vi "Apply Surface.vi"(5 "x":i32, 7 "y":i32, 8 "error in":errorcluster, 10 "Destination Pointer":u32, 11 "Source Pointer":u32) -> (0 "error out":errorcluster)   [LabVIEW 2015]
uses:
  Controls/Rectangle.ctl
  LibSDL2.lvlib
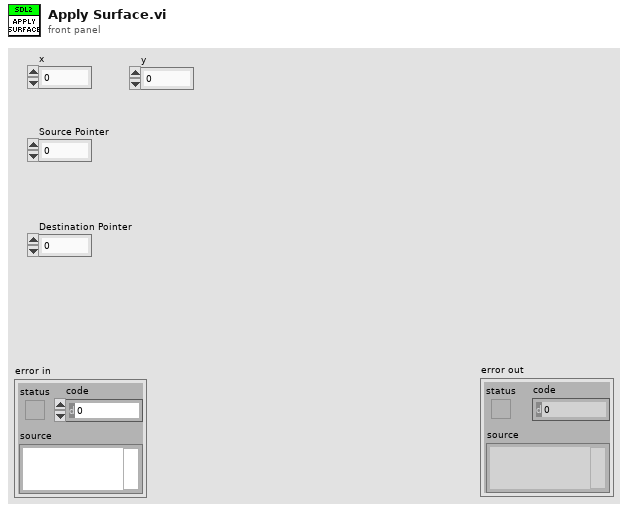
[diagram p1: front panel]
types:
  T1 = typedef "LibSDL2.lvlib/Rectangle.ctl" = cluster{"x":i32, "y":i32, "Width":i32, "Height":i32}
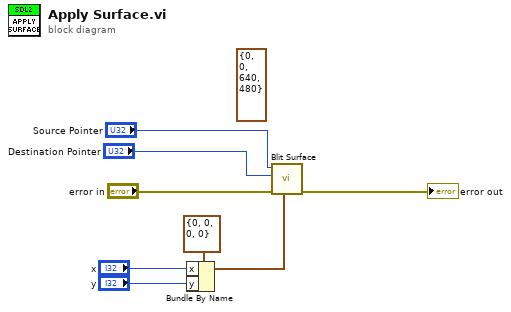
[diagram p0: block diagram]
diagram:
  (unwired) T1 {"x"=0, "y"=0, "Width"=640, "Height"=480} ("Source Rectangle")
  n1 = Bundle By Name(cluster=T1 {"x"=0, "y"=0, "Width"=0, "Height"=0} ("Rectangle"), "x"="x", "y"="y") -> (w2:T1)
  n2 = call "Blit Surface.vi"("Destination Rectangle Pointer"=w2, "error in"="error in", "Source Rectangle Pointer"="Destination Pointer", "Source Surface Pointer"="Source Pointer") -> ("error out"=→"error out":errorcluster)  [unwired: 6 in, 1 out]
